vi "FindnReplace.vi"(8 "Front Panel":refnum<vi>, 11 "Python Code":refnum<vi>) -> ()   [LabVIEW 2022 SP3]
uses:
  <vilib>/Utility/miscctls.llb/LVSelectionTypeDef.ctl
panel:
  out "last selection":T1
  in  "Replace?":bool
  in  "forward":bool
  in  "back":bool
  in  "Replace":string
  in  "Find":string
  out "found":string
  out "element":i32
  out "# hits":i32
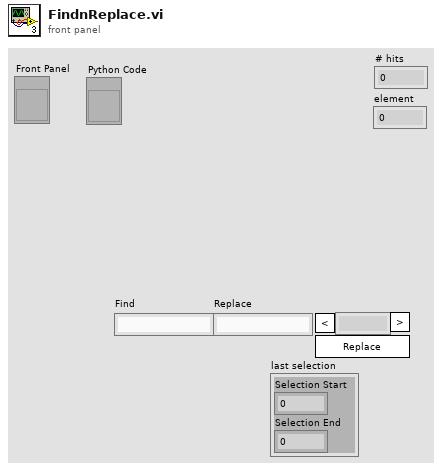
[diagram p1: front panel]
types:
  T1 = typedef "LVSelectionTypeDef.ctl" = cluster{"Selection Start":u32, "Selection End":u32}
  T2 = cluster{"Find":string, "Replace":string, "back":bool, "forward":bool, "searcn":bool, "junk":string}
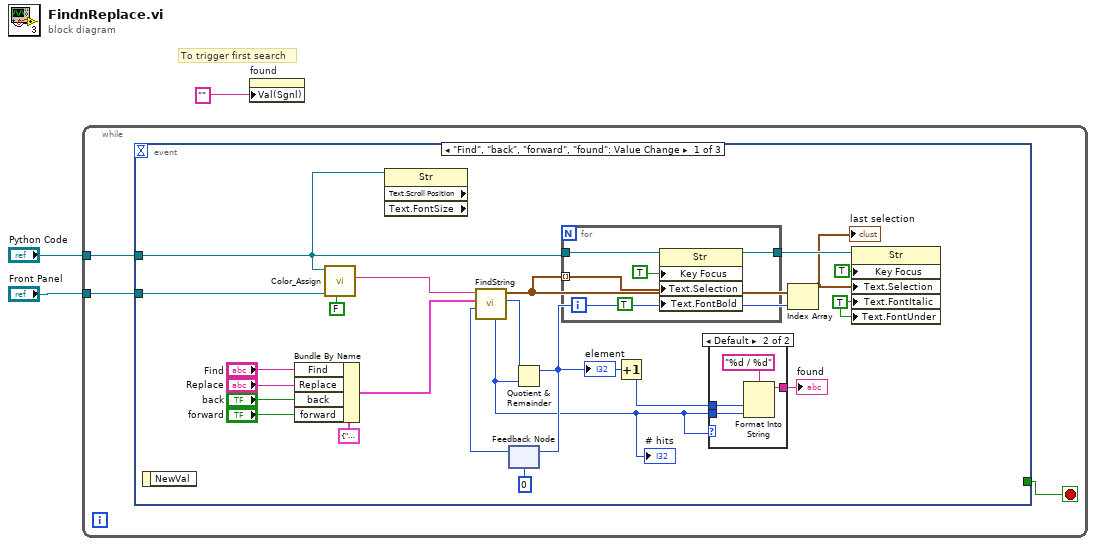
[diagram p0: block diagram]
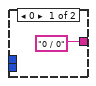
[diagram p2: hidden frame]
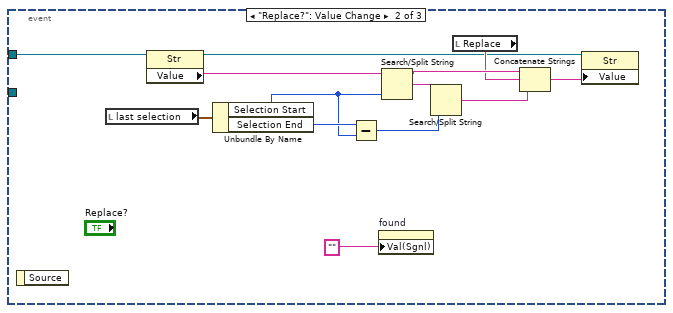
[diagram p3: hidden frame]
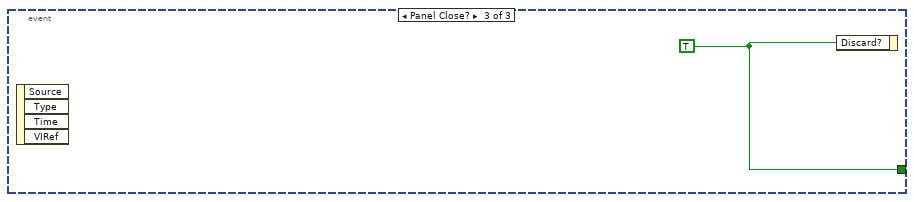
[diagram p4: hidden frame]
diagram:
  # "To trigger first search"
  n1 = while {
    tunnel: "Python Code" -> [w5]
    tunnel: "Front Panel" -> [w4]
    stop <- w6 stop-if-true
    n2 = event shown="[0] \"Find\", \"back\", \"forward\", \"found\": Value Change" {
      selector: _ -> [_ _ _]
      dyn-events: _ -> [_ _ _]
      timeout: _ -> [_ _ _]
      tunnel: [_ _ w52] -> w6
      tunnel: w5 -> [w7 w51 _]
      tunnel: w4 -> [w10 _ _]
      event "Find", "back", "forward", "found": Value Change {
        w11 = TRUE ("Text.Font:Italic")
        n3 = event-data() -> ()  [unwired: 1 in, 1 out]
        n4 = Bundle By Name(cluster=T2 {"Find"="hub.dis", "Replace"="", "back"=FALSE, "forward"=FALSE, "searcn"=FALSE, "junk"=""} ("FnR"), "Find"="Find", "Replace"="Replace", "back"="back", "forward"="forward") -> (w17:T2)
        n5 = call "Color_Assign.vi"("Add Spaces?"=FALSE, "Front Panel"=w10, "Code"=w7) -> ("Value"=w22:string)  [unwired: 8 in]
        n6 = property on="Property Node" class="Str" props=["Text", "Scroll Position", "Text", "FontSize"](reference=w7) -> ()  [unwired: 1 in, 4 out]
        n7 = feedback #1(0) -> (w28:i32)
        n8 = call "FindString.vi"("offset past match in"=w28, "FnR"=w17, "String"=w22) -> ("offset past match out"=w25:i32, "Array"=w14:T1[], "# hits"=w8:i32)  [unwired: 6 in]
        "# hits" <- w8
        n9 = Quotient & Remainder(x=w25, y=w8) -> (x-y*floor(x/y)=w13:i32)  [unwired: 1 out]
        "element" <- w13
        n10 = feedback-in #1(w13) -> ()
        n11 = for {
          tunnel: w14 -> [w35] mode=indexing
          tunnel: w7 -> [w37]
          tunnel: [w34] -> w16
          n12 = property on="Property Node" class="Str"(reference=w37, "Key Focus"=TRUE, "Text.Selection"=w35, "Text.FontBold"=TRUE ("Text.Font:Bold")) -> (reference out=w34:refnum<vi>)  [unwired: 1 in, 1 out]
        }
        n13 = Increment(x=w13) -> (x+1=w24:i32)
        n14 = case shown="Default" w8 {
          tunnel: w8 -> [_ w32]
          tunnel: ["0 / 0" ("format string") w31] -> w26
          tunnel: w24 -> [_ w30]
          frame 0 {
          }
          frame Default {
            n15 = Format Into String(format string="%d / %d", w30, w32) -> (resulting string=w31:string)  [unwired: 2 in, 1 out]
          }
        }
        "found" <- w26
        n16 = Index Array(array=w14, index=w13) -> (element=w12:T1)
        "last selection" <- w12
        n17 = property on="Property Node" class="Str"(reference=w16, "Key Focus"=TRUE, "Text.Selection"=w12, "Text.FontItalic"=w11, "Text.FontUnder"=w11) -> ()  [unwired: 1 in, 2 out]
      }
      event "Replace?": Value Change {
        n18 = event-data() -> ()  [unwired: 1 in, 1 out]
        n19 = local read "last selection"() -> (w50:T1)
        n20 = property on="Property Node" class="Str"(reference=w51) -> (reference out=w41:refnum<vi>, "Value"=w49:string)  [unwired: 1 in, 1 out]
        n21 = Unbundle By Name(w50) -> ("Selection Start"=w46:u32, "Selection End"=w47:u32)
        n22 = Subtract(x=w47, y=w46) -> (x-y=w45:u32)
        n23 = property on="found" class="Str"("Val(Sgnl)"="" ("Value (Signaling)")) -> ()  [unwired: 2 in, 2 out]
        n24 = Search/Split String(string=w49, offset (0)=w46) -> (substring before match=w44:string, match + rest of string=w48:string)  [unwired: 1 in, 1 out]
        n25 = Search/Split String(string=w48, offset (0)=w45) -> (match + rest of string=w43:string)  [unwired: 1 in, 2 out]
        n26 = local read "Replace"() -> (w42:string)
        n27 = Concatenate Strings(w44, w42, w43) -> (w40:string)
        n28 = property on="Property Node" class="Str"(reference=w41, "Value"=w40) -> ()  [unwired: 1 in, 2 out]
      }
      event Panel Close? {
        w52 = TRUE
        n29 = event-data() -> ()  [unwired: 1 in, 4 out]
        n30 = event-data("Discard?"=w52) -> ()  [unwired: 1 in, 1 out]
      }
    }
  }
  n31 = property on="found" class="Str"("Val(Sgnl)"="" ("Value (Signaling)")) -> ()  [unwired: 2 in, 2 out]
